vi "test swap.vi"() -> ()   [LabVIEW 2014]
panel:
  out "Boolean array 2":bool[](array[boolean])
  in  "Boolean array":bool[](array[boolean])
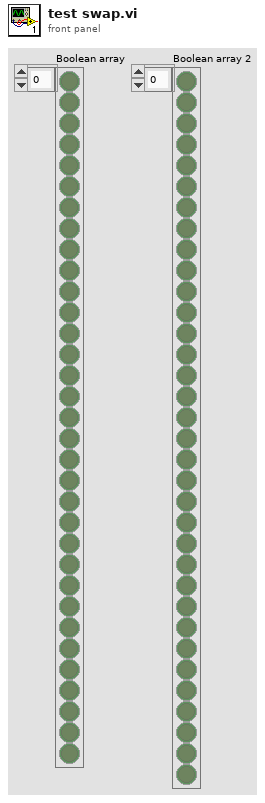
[diagram p1: front panel]
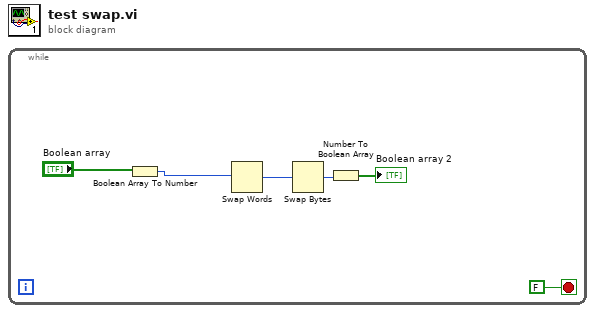
[diagram p0: block diagram]
diagram:
  n1 = while {
    stop <- FALSE stop-if-true
    n2 = Boolean Array To Number(Boolean array="Boolean array") -> (number=w4:u32)
    n3 = Swap Words(1:w4) -> (0:w6:u32)
    n4 = Swap Bytes(anything=w6) -> (byte swapped=w3:u32)
    n5 = Number To Boolean Array(number=w3) -> (Boolean array=→"Boolean array 2":bool[])
  }
